vi "Write WriteTimeout.vi"(8 "error in (no error)":errorcluster, 10 "WriteTimeout":i32=5000, 11 "ServerConfig in":refnum<class "ServerConfig.lvclass">) -> (0 "error out":errorcluster, 3 "ServerConfig out":refnum<class "ServerConfig.lvclass">)   [LabVIEW 2022 SP3, in "TcpServer.lvlib" / "ServerConfig.lvclass"]
uses:
  ServerConfig.lvclass
  ServerConfig.lvclass/ServerConfig.ctl
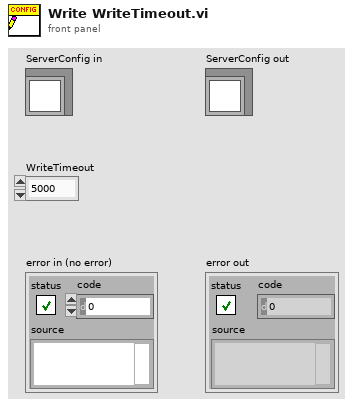
[diagram p1: front panel]
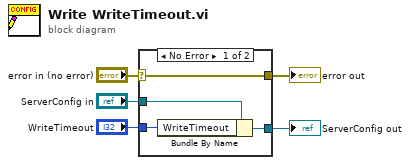
[diagram p0: block diagram]
diagram:
  n1 = case shown="No Error" "error in (no error)" {
    selector: "error in (no error)" -> [w9 w10]
    tunnel: [w9 w10] -> w4
    tunnel: [w7 w11] -> w2
    tunnel: "ServerConfig in" -> [w8 w11]
    tunnel: "WriteTimeout" -> [w6 _]
    frame No Error {
      n2 = Bundle By Name(cluster=w8, "WriteTimeout"=w6) -> (w7:refnum<class "ServerConfig.lvclass">)
    }
    frame Error {
    }
  }
  "error out" <- w4
  "ServerConfig out" <- w2
